vi "CSM - Replace Marks in Messages.vi"(5 "States With Replace Token":string, 7 "<param>":string, 9 "<target>":string, 12 "<1>":string, 13 "<2>":string) -> (6 "States":string)   [LabVIEW 2017, in "Communicable State Machine.lvlib"]
doc: "Facilitates editing multiple CSM message strings by providing a batch replacement function for marks. There are four marks that can be replaced:\n- `<param>` mark: Usually represents the same argument.\n- `<target>` mark: Usually represents the same target.\n- `<1>` mark: Represents custom mark 1.\n- `<2>` mark: Represents custom mark 2.\n\n<b>Example</b>: The terminal `<target>` is connected to the string `DAQDevice`. The <b>States with Replace Token</b> string is:\n\n text\n Initialize -@ <target>\n Configure -@ <target>\n Read -@ <target>\n Close -@ <target>\n\nThe <b>States</b> output is:\n\n text\n Initialize -@ DAQDevice\n Configure -@ DAQDevice\n Read -@ DAQDevice\n Close -@ DAQDevice\n\n\n> [!NOTE] <b>Message Building API</b>\n>\n> This type of API is only used to concatenate message strings and does not send messages directly. The strings need to be merged into the CSM state queue, and the messages will be sent and the operation executed within the Parse State Queue++ VI. If you are familiar with CSM rules, you do not need to use this type of API. You can type the corresponding message string or operation string directly into the string.\n\n\n-- <b>Controls</b> --\n- <b>States with Replace Token</b>: CSM state string with replacement marks.\n- <b><param></b>: `<param>` mark, which usually represents the same argument.\n- <b><target></b>: `<target>` mark, which usually represents the same target.\n- <b><1></b>: Custom mark 1.\n- <b><2></b>: Custom mark 2.\n\n-- <b>Indicators</b> --\n- <b>States</b>: State string after replacement."
uses:
  Communicable State Machine.lvlib
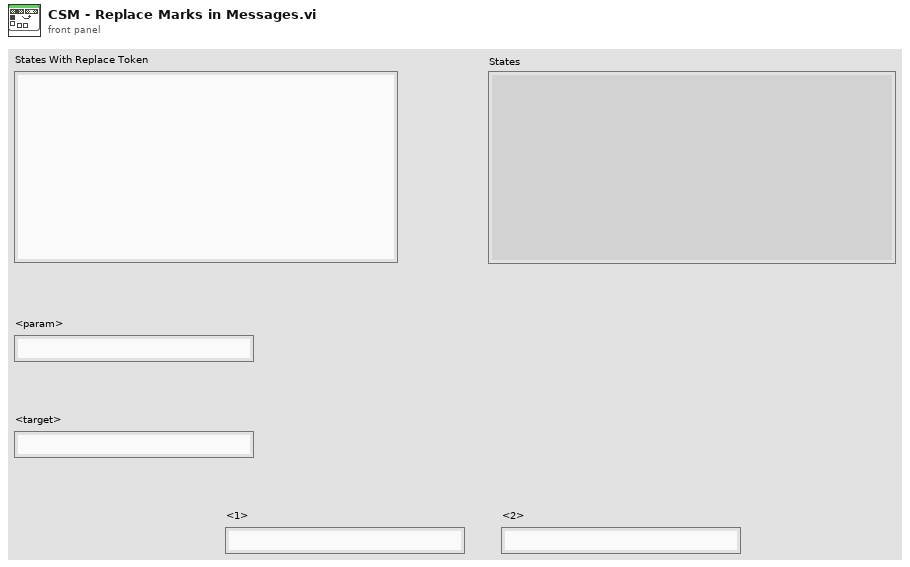
[diagram p1: front panel]
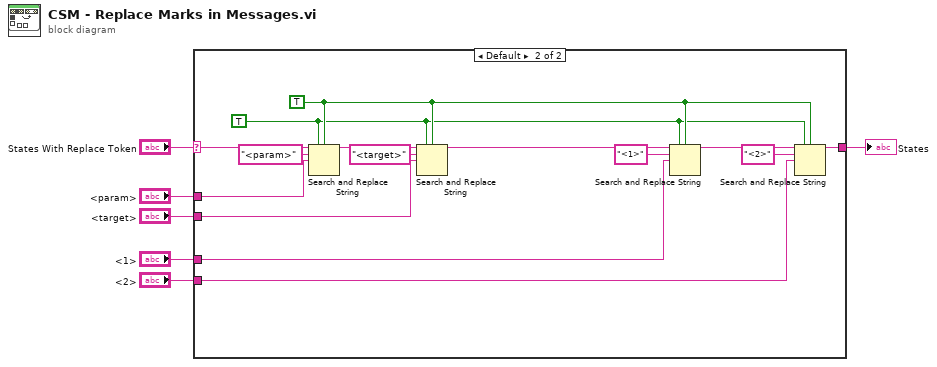
[diagram p0: block diagram]
diagram:
  n1 = case shown="Default" "States With Replace Token" {
    selector: "States With Replace Token" -> [w7 w22]
    tunnel: "<param>" -> [_ w21]
    tunnel: "<target>" -> [_ w20]
    tunnel: [w7 w12] -> w5
    tunnel: "<2>" -> [_ w9]
    tunnel: "<1>" -> [_ w8]
    frame "" {
    }
    frame Default {
      w11 = TRUE ("ignore case? (F)")
      w10 = TRUE ("replace all? (F)")
      n2 = Search and Replace String(replace all?=w10, case sensitive?=w11, input string=w22, search string="<param>", replace string=w21) -> (result string=w19:string)  [unwired: 3 in, 3 out]
      n3 = Search and Replace String(replace all?=w10, case sensitive?=w11, input string=w19, search string="<target>", replace string=w20) -> (result string=w18:string)  [unwired: 3 in, 3 out]
      n4 = Search and Replace String(replace all?=w10, case sensitive?=w11, input string=w18, search string="<1>", replace string=w8) -> (result string=w13:string)  [unwired: 3 in, 3 out]
      n5 = Search and Replace String(replace all?=w10, case sensitive?=w11, input string=w13, search string="<2>", replace string=w9) -> (result string=w12:string)  [unwired: 3 in, 3 out]
    }
  }
  "States" <- w5
